vi "menu-ReplaceSeperatorWith---.vi"(11 "Array in":T1[](array[typedef])) -> (3 "Array out":T1[](array[typedef]))   [LabVIEW 2017, in "menu-operation.lvlib"]
uses:
  menu-operation.lvlib
  <resource>/Framework/Providers/API/mxLvMenuItem.ctl
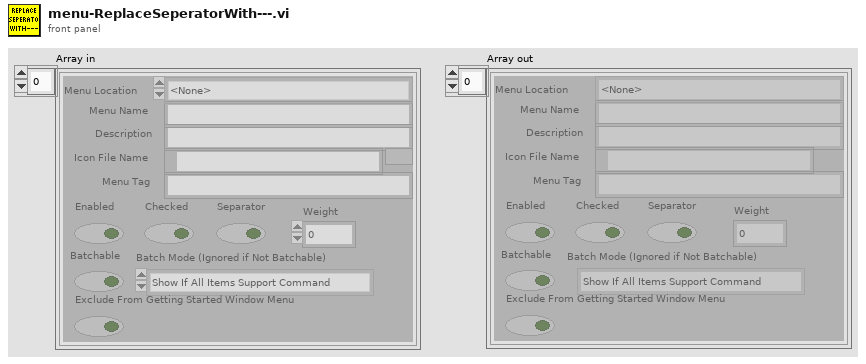
[diagram p1: front panel]
types:
  T1 = typedef "mxLvMenuItem.ctl" = cluster{"Menu Name":string, "Description":string, "Icon File Name":path, "Menu Tag":string, "Enabled":bool, "Checked":bool, "Separator":bool, "Batchable":bool, "Weight":i32, "Batch Mode (Ignored if Not Batchable)":enum32{"Show If All Items Support Command", "Show If Any Items Support Command"}, "Menu Location":enum32{"<None>", "Project", "Project / Build Specifications", "Tools", "Tools / Source Control", "Tools / Real-Time Module", "Help"}, "Exclude From Getting Started Window Menu":bool}
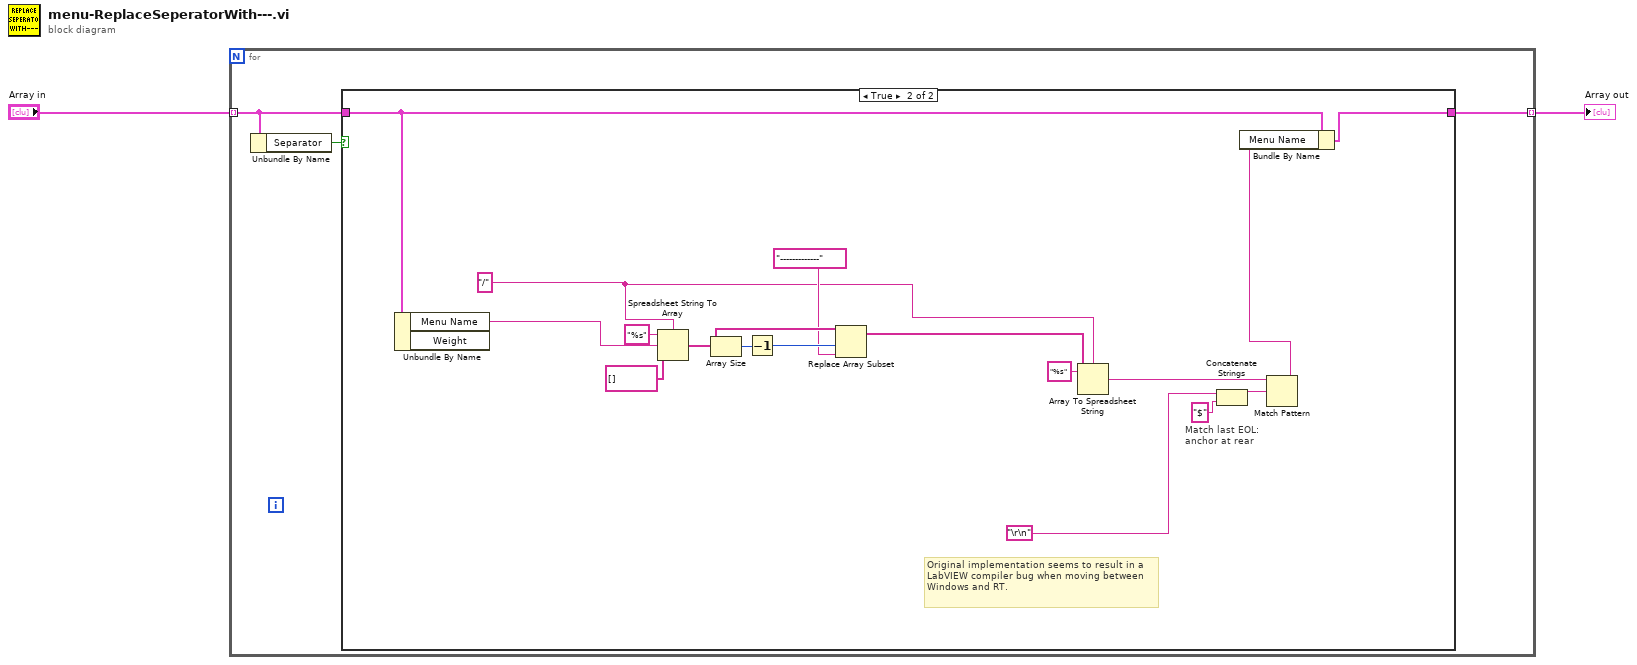
[diagram p0: block diagram]
diagram:
  n1 = for {
    tunnel: "Array in" -> [w4] mode=indexing
    tunnel: [w5] -> w1 mode=indexing
    n2 = Unbundle By Name(w4) -> ("Separator"=w3:bool)
    n3 = case shown="True" w3 {
      tunnel: [w6 w23] -> w5
      tunnel: w4 -> [w6 w15]
      frame False {
      }
      frame True {
        w16 = "/" ("delimiter (Tab)")
        # "Original implementation seems to result in a LabVIEW compiler bug when moving between Windows and RT."
        # "Match last EOL:\nanchor at rear"
        n4 = Unbundle By Name(w15) -> ("Menu Name"=w22:string)  [unwired: 1 out]
        n5 = Spreadsheet String To Array(delimiter (Tab)=w16, format string="%s", spreadsheet string=w22, array type (2D Dbl)=string[] [] ("Array of Strings")) -> (array=w20:string[])
        n6 = Array Size(array=w20) -> (size(s)=w21:i32)
        n7 = Decrement(x=w21) -> (x-1=w19:i32)
        n8 = Replace Array Subset(array=w20, new element="-------------" ("delimiter (Tab)"), index=w19) -> (w17:string[])
        n9 = Array To Spreadsheet String(delimiter (Tab)=w16, array=w17, 3:"%s" ("format string")) -> (spreadsheet string=w10:string)
        n10 = Concatenate Strings("\r\n", "$" ("Substring")) -> (w9:string)
        n11 = Match Pattern(string=w10, regular expression=w9) -> (before substring=w14:string)  [unwired: 1 in, 3 out]
        n12 = Bundle By Name(cluster=w15, "Menu Name"=w14) -> (w23:T1)
      }
    }
  }
  "Array out" <- w1
